vi "GetFiducialMarkTemplate (SubVI).vi"(8 "error in (no error)":errorcluster, 9 "Module fiducial marker":T3, 10 "Sensor Pattern":T2(ring)=enum."ATLAS12", 11 "Templates path":path=path "C:/Users/Aerotech/Documents/BNL_ThermomechanicalStave") -> (0 "error out":errorcluster, 1 "Template out 2":T4(plugin-control), 2 "Mark string":string, 3 "Template out":T4(plugin-control))   [LabVIEW 2016]
uses:
  Utils/Controls/All_Enums/Enum_TypeDef_FidMarkers.ctl
panel:
  in  "Tab Control":T1(tab)
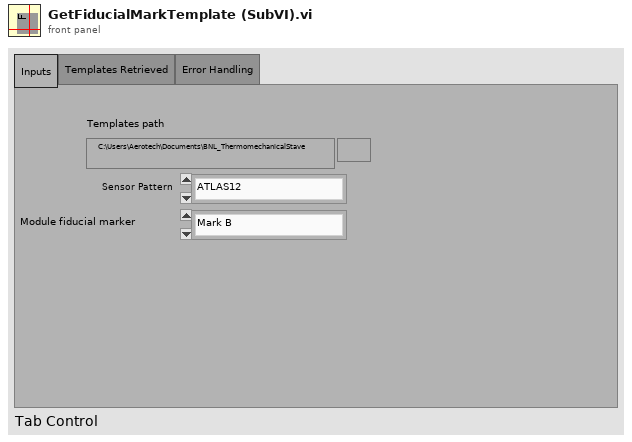
[diagram p1: front panel]
types:
  T1 = enum32{"Inputs", "Templates Retrieved", "Error Handling"}
  T2 = enum16{"ATLAS07", "ATLAS12", "ATLAS12Slim", "ATLAS17LS"}
  T3 = typedef "Enum_TypeDef_FidMarkers.ctl" = enum16{"Mark B", "Mark C", "Bias Ring Corner", "Mark I (Slim/17)", "Mark E (Slim/17)", "Mark F (Slim/17)", "Mark G (Slim/17)", "Mark A (12)", "Kapton Spacers"}
  T4 = typedef "IMAQ Image.ctl" = refnum<image>
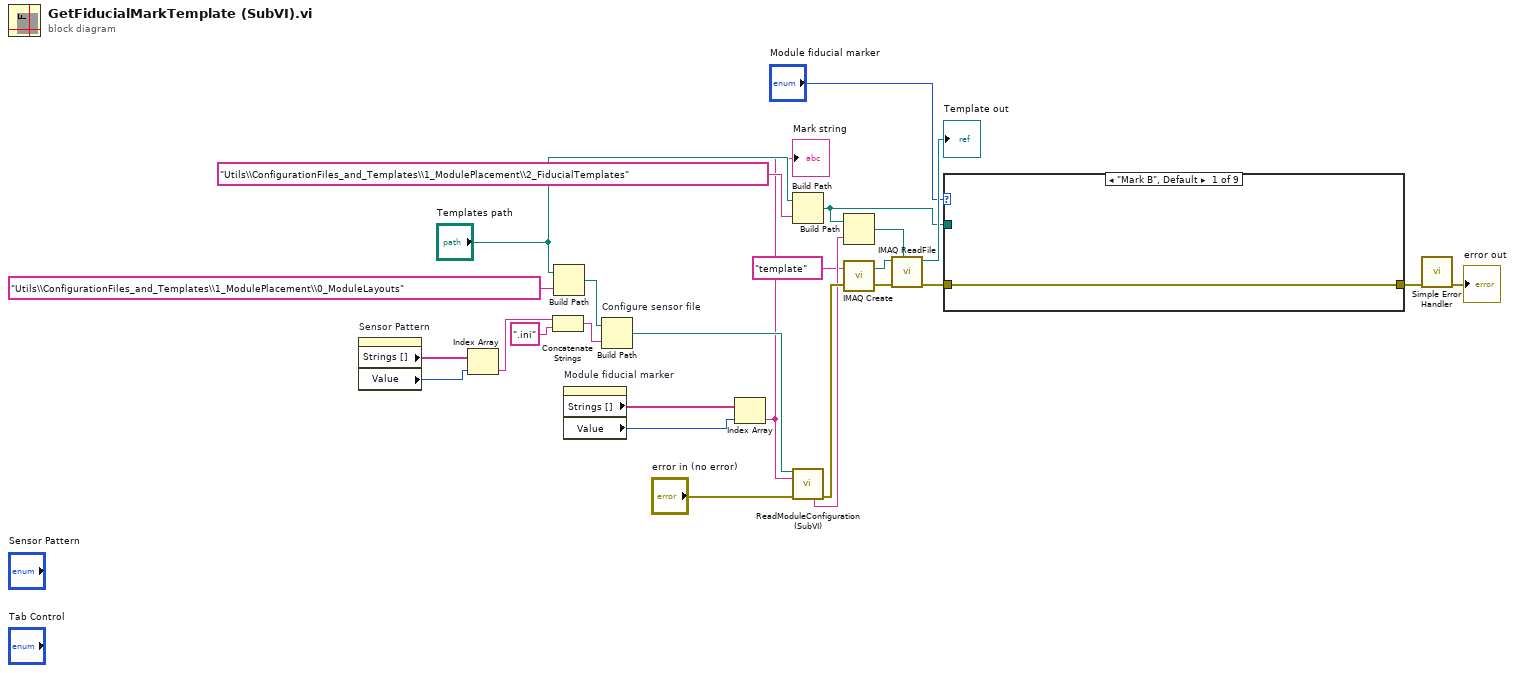
[diagram p0: block diagram]
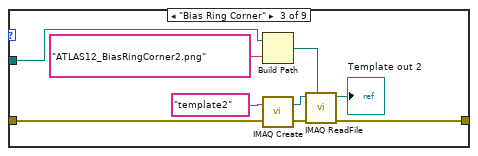
[diagram p3: hidden frame]
diagram:
  n1 = property on="Sensor Pattern" class="Enum (strict)"() -> ("Strings []"=w7:string[], "Value"=w6:T2)  [unwired: 2 in, 2 out]
  n2 = Index Array(array=w7, index=w6) -> (element=w10:string)
  n3 = Concatenate Strings(w10, ".ini" ("string")) -> (w8:string)
  n4 = Build Path(base path="Templates path", name or relative path="Utils\\ConfigurationFiles_and_Templates\\1_ModulePlacement\\0_ModuleLayouts") -> (appended path=w5:path)
  n5 = property on="Module fiducial marker" class="Enum (strict)"() -> ("Strings []"=w2:string[], "Value"=w3:T3)  [unwired: 2 in, 2 out]
  n6 = Build Path "Configure sensor file"(base path=w5, name or relative path=w8) -> (appended path=w4:path)
  n7 = Index Array(array=w2, index=w3) -> (element=w1:string)
  "Mark string" <- w1
  n8 = Build Path(base path="Templates path", name or relative path="Utils\\ConfigurationFiles_and_Templates\\1_ModulePlacement\\2_FiducialTemplates") -> (appended path=w11:path)
  n9 = call "ReadModuleConfiguration (SubVI).vi"("Module configuration file path"=w4, "Fiducial Mark"=w1, "error in (no error)"="error in (no error)") -> ("Template filename"=w24:string, "error out"=w26:errorcluster)  [unwired: 6 in, 5 out]
  n10 = Build Path(base path=w11, name or relative path=w24) -> (appended path=w15:path)
  n11 = call "IMAQ Create"("Image Name"="template", "error in (no error)"=w26) -> ("New Image"=w18:T4, "error out"=w19:errorcluster)  [unwired: 3 in]
  n12 = call "IMAQ ReadFile"("File Path"=w15, "error in (no error)"=w19, "Image"=w18) -> ("error out"=w13:errorcluster, "Image Out"=→"Template out":T4)  [unwired: 4 in, 3 out]
  n13 = case shown="\"Mark B\", Default" "Module fiducial marker" {
    tunnel: w13 -> [w27 w28 w35 w38 w39 w40 w41 w42 w43]
    tunnel: [w27 w28 w34 w38 w39 w40 w41 w42 w43] -> w12
    tunnel: w11 -> [_ _ w31 _ _ _ _ _ _]
    frame "Mark B", Default {
    }
    frame "Mark C" {
    }
    frame "Bias Ring Corner" {
      n14 = Build Path(base path=w31, name or relative path="ATLAS12_BiasRingCorner2.png") -> (appended path=w29:path)
      n15 = call "IMAQ Create"("Image Name"="template2", "error in (no error)"=w35) -> ("New Image"=w33:T4, "error out"=w36:errorcluster)  [unwired: 3 in]
      n16 = call "IMAQ ReadFile"("File Path"=w29, "error in (no error)"=w36, "Image"=w33) -> ("error out"=w34:errorcluster, "Image Out"=→"Template out 2":T4)  [unwired: 4 in, 3 out]
    }
    frame "Mark I (Slim/17)" {
    }
    frame "Mark E (Slim/17)" {
    }
    frame "Mark F (Slim/17)" {
    }
    frame "Mark G (Slim/17)" {
    }
    frame "Mark A (12)" {
    }
    frame "Kapton Spacers" {
    }
  }
  n17 = call <vilib>:"Simple Error Handler.vi"("error in (no error)"=w12) -> ("error out"=→"error out":errorcluster)  [unwired: 4 in, 4 out]
